vi "SetFPref.vi"(8 "error in (no error)":errorcluster, 10 "FPref":T1, 11 "reference in":refnum<class "XYgraph.lvclass">) -> (0 "error out":errorcluster, 3 "reference out":refnum<class "XYgraph.lvclass">)   [LabVIEW 2019, in "XYgraph.lvclass"]
uses:
  XYgraph.lvclass
  XY graph ref.ctl
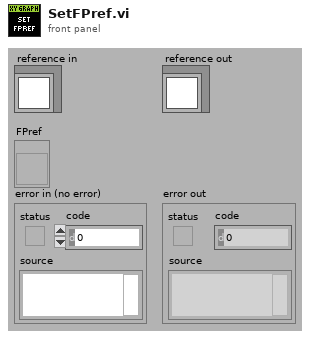
[diagram p1: front panel]
types:
  T1 = typedef "XYgraph.lvclass/XY graph ref.ctl" = refnum<vi>
  T2 = typedef "XYgraph.lvclass/ObjectAttributesRef.ctl" = refnum<data-value>
  T3 = typedef "XYgraph.lvclass/ObjectAttributes.ctl" = cluster{"FPref":T1, "MyAttribute":dbl, "X multiplier":dbl, "Y multiplier":dbl, "X Scale name":string, "Y Scale name":string, "Fcurve metadata":T4, "Fcurve":refnum<class "Fcurve.lvclass">}
  T4 = typedef "Fcurve.lvclass/Metadata.ctl" = cluster{"dt (us)":dbl, "Dec Factor":dbl, "Z piezo Sensitivity (nm/V)":dbl, "K (N/m)":dbl, "Sp (V)":dbl, "Contact (ms)":dbl, "Zpos contact":dbl, "Vel_app (nm/s)":dbl, "Vel_ret (nm/s)":dbl, "deltaV (nm)":dbl, "Def_V0 (v)":dbl, "Piezo gain":dbl, "invOLS (nm/V)":dbl}
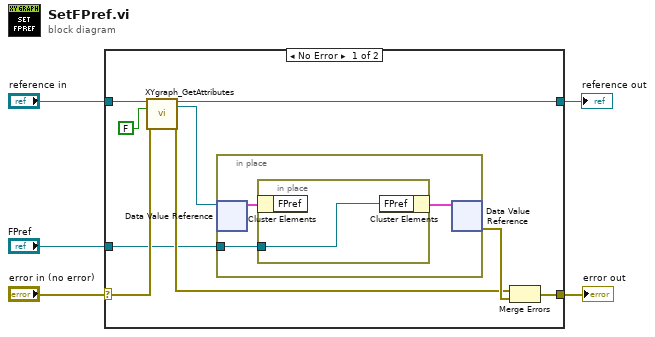
[diagram p0: block diagram]
diagram:
  n1 = case shown="No Error" "error in (no error)" {
    selector: "error in (no error)" -> [w14 w20]
    tunnel: [w8 w20] -> w4
    tunnel: [w13 w19] -> w2
    tunnel: "reference in" -> [w12 w19]
    tunnel: "FPref" -> [w6 _]
    frame No Error {
      n2 = call "XYgraph_GetAttributes.vi"("reference in"=w12, "return data? (T)"=FALSE, "error in (no error)"=w14) -> ("reference out"=w13:refnum<class "XYgraph.lvclass">, "attributes ref"=w7:T2, "error out"=w9:errorcluster)  [unwired: 13 in, 1 out]
      n3 = in-place {
        in-place-border: w6 -> [w15]
        n4 = in-place-dvr #1(w7) -> (w16:T3)  [unwired: 1 out]
        n5 = in-place {
          in-place-border: w15 -> [w18]
          n6 = in-place-cluster #2(w16) -> ()  [unwired: 1 out]
          n7 = in-place-cluster #2("FPref"=w18) -> (w17:T3)
        }
        n8 = in-place-dvr #1(w17) -> (w10:errorcluster)  [unwired: 1 out]
      }
      n9 = Merge Errors(w9, w10) -> (w8:errorcluster)
    }
    frame Error {
    }
  }
  "error out" <- w4
  "reference out" <- w2
